vi "Read Name.vi"(11 "Build Package Item in":refnum<class "Build Package Item.lvclass">) -> (2 "Name":string)   [LabVIEW 2019, in "VIPM.lvlib" / "Build Package Item.lvclass"]
doc: "Returns the name of the solution item.\n----\nCopyright: MGI 2017\nAuthor: Derek Trepanier"
uses:
  Build Package Item.lvclass
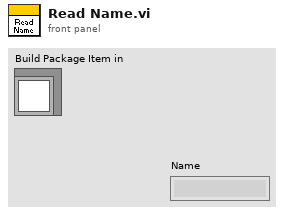
[diagram p1: front panel]
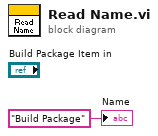
[diagram p0: block diagram]
diagram:
  "Name" <- "Build Package" ("Name")
